vi "USB.Check Device using Service, PID, and VID.vi"(6 "Check for Multiple":bool, 8 "error in":errorcluster, 9 "PID":string="2603", 10 "VID":string="28DE", 11 "Service":string="usbaudio") -> (0 "error out":errorcluster, 2 "Qty":i32, 3 "Found":bool)   [LabVIEW 2018]
uses:
  <vilib>/registry/registry.llb/Registry RtKey.ctl
  <vilib>/registry/registry.llb/Registry SAM.ctl
panel:
  out "String/Binary data":string[](array[string])
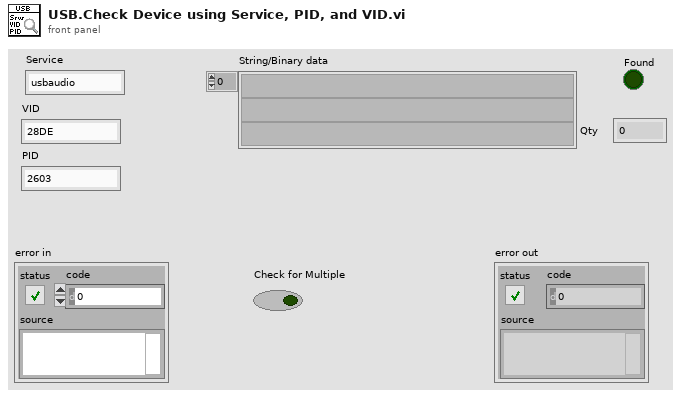
[diagram p1: front panel]
types:
  T1 = typedef "Registry SAM.ctl" = enum32{"KEY_QUERY_VALUE", "KEY_SET_VALUE", "KEY_CREATE_SUB_KEY", "KEY_ENUMERATE_SUB_KEYS", "KEY_NOTIFY", "KEY_CREATE_LINK", "KEY_READ", "KEY_WRITE", "KEY_ALL_ACCESS", "KEY_READ | KEY_WRITE"}
  T2 = typedef "Registry RtKey.ctl" = enum32{"HKEY_CLASSES_ROOT", "HKEY_CURRENT_USER", "HKEY_LOCAL_MACHINE", "HKEY_USERS", "HKEY_PERFORMANCE_DATA", "HKEY_CURRENT_CONFIG", "HKEY_DYN_DATA"}
  T3 = typedef "Registry refnum.ctl" = refnum<k1>
  T4 = cluster{"numValues":i32, "maxValueNameLen":i32, "maxValueDataLen":i32}
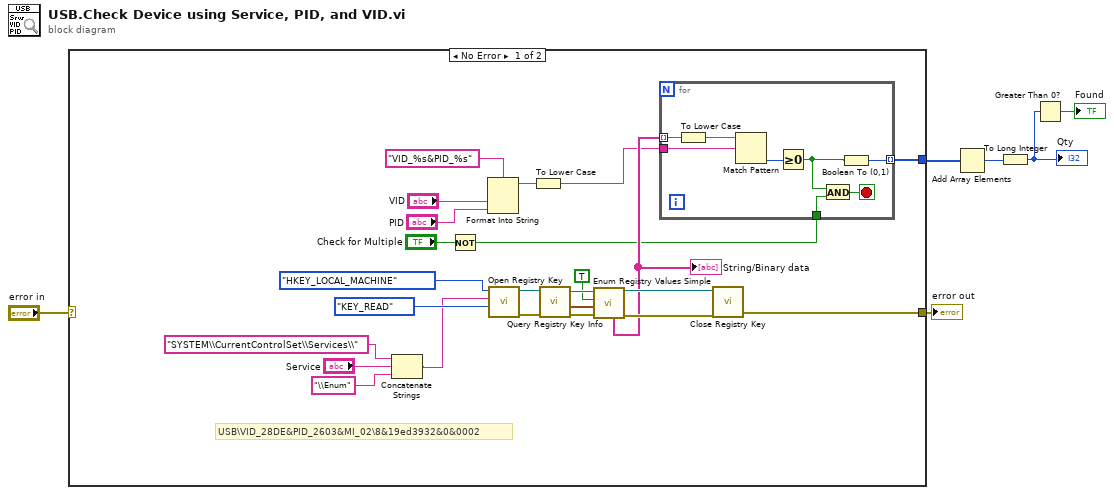
[diagram p0: block diagram]
diagram:
  n1 = case shown="No Error" "error in" {
    selector: "error in" -> [_ w39]
    tunnel: [w20 w39] -> w6
    tunnel: [w13 _] -> w4
    frame No Error {
      # "USB\\VID_28DE&PID_2603&MI_02\\8&19ed3932&0&0002"
      n2 = Concatenate Strings("SYSTEM\\CurrentControlSet\\Services\\", "Service", "\\Enum") -> (w9:string)
      n3 = Not(x="Check for Multiple") -> (.not. x?=w7:bool)
      n4 = Format Into String(format string="VID_%s&PID_%s", "VID", "PID") -> (resulting string=w15:string)  [unwired: 2 in, 1 out]
      n5 = call <vilib>:"Open Registry Key.vi"("security access mask (KEY_READ | KEY_WRITE)"=Registry_SAM."KEY_READ", "subkey"=w9, "root key (HKEY_LOCAL_MACHINE)"=Registry_RtKey."HKEY_LOCAL_MACHINE") -> ("error out"=w27:errorcluster, "refnum out"=w28:T3)  [unwired: 1 in, 6 out]
      n6 = To Lower Case(string=w15) -> (all lower case string=w14:string)
      n7 = call <vilib>:"Query Registry Key Info.vi"("error in (no error)"=w27, "refnum"=w28) -> ("error out"=w26:errorcluster, "value info"=w24:T4, "refnum out"=w25:T3)  [unwired: 7 out]
      n8 = call <vilib>:"Enum Registry Values Simple.vi"("error in (no error)"=w26, "value info"=w24, "retrieve data? (F)"=TRUE, "refnum"=w25) -> ("error out"=w21:errorcluster, "refnum out"=w22:T3, "String/Binary data"=w19:string[])  [unwired: 2 in, 3 out]
      "String/Binary data" <- w19
      n9 = for {
        tunnel: w19 -> [w38] mode=indexing
        tunnel: [w32] -> w13 mode=indexing
        tunnel: w14 -> [w35]
        tunnel: w7 -> [w33]
        stop <- w34 stop-if-true
        n10 = To Lower Case(string=w38) -> (all lower case string=w37:string)
        n11 = Match Pattern(string=w37, regular expression=w35) -> (offset past match=w36:i32)  [unwired: 1 in, 3 out]
        n12 = Greater Or Equal To 0?(x=w36) -> (x >= 0?=w31:bool)
        n13 = And(x=w31, y=w33) -> (x .and. y?=w34:bool)
        n14 = Boolean To (0,1)(Boolean=w31) -> (0, 1=w32:i16)
      }
      n15 = call <vilib>:"Close Registry Key.vi"("error in (no error)"=w21, "refnum"=w22) -> ("error out"=w20:errorcluster)  [unwired: 5 out]
    }
    frame Error {
    }
  }
  "error out" <- w6
  n16 = Add Array Elements(numeric array=w4) -> (sum=w3:i16)
  n17 = To Long Integer(number=w3) -> (32bit integer=w2:i32)
  "Qty" <- w2
  n18 = Greater Than 0?(x=w2) -> (x > 0?=→"Found":bool)
